vi "Read Active.vi"(8 "error in (no error)":errorcluster, 11 "DAQmxTask in":refnum<class "DAQmxTask.lvclass">) -> (0 "error out":errorcluster, 2 "Active?":bool, 3 "DAQmxTask out":refnum<class "DAQmxTask.lvclass">)   [LabVIEW 2018, in "DAQmxTask.lvclass"]
uses:
  DAQmxTask.lvclass
  DAQmxTask.lvclass/DAQmxTask.ctl
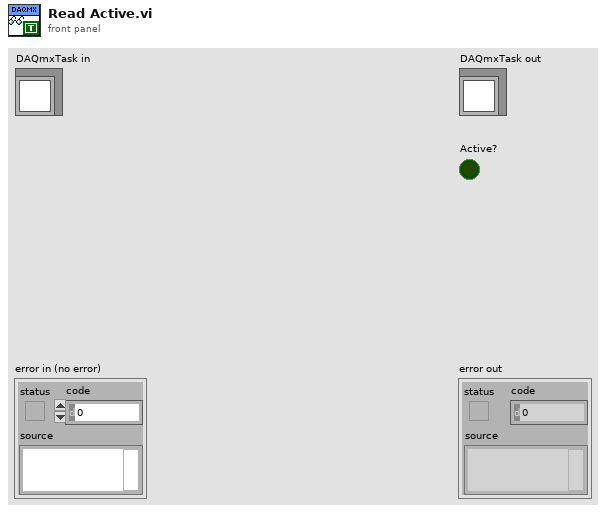
[diagram p1: front panel]
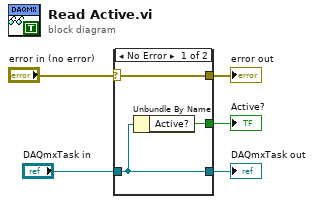
[diagram p0: block diagram]
diagram:
  n1 = case shown="No Error" "error in (no error)" {
    selector: "error in (no error)" -> [w8 w9]
    tunnel: [w8 w9] -> w4
    tunnel: [w7 w10] -> w2
    tunnel: "DAQmxTask in" -> [w7 w10]
    tunnel: [w6 _] -> w1
    frame No Error {
      n2 = Unbundle By Name(w7) -> ("Active?"=w6:bool)
    }
    frame Error {
    }
  }
  "error out" <- w4
  "DAQmxTask out" <- w2
  "Active?" <- w1
